vi "Set Modules.vi"(6 "wait for reply (T)":bool=TRUE, 8 "error in (no error)":errorcluster, 10 "Module Paths":path[](array[path])=[path "Modules/Dummie"]) -> (0 "error out":errorcluster, 1 "timed out?":bool)   [LabVIEW 2022 SP3, in "UI Manager.lvlib"]
doc: "Lets UI know which modules are loaded so it can register for broadcast events\n____\nHAMPEL SOFTWARE ENGINEERING v2.6.0 (2023-12-19 10:54)"
uses:
  UI Manager.lvlib
  Set Modules Argument--cluster.ctl
  Set Modules (Reply Payload)--cluster.ctl
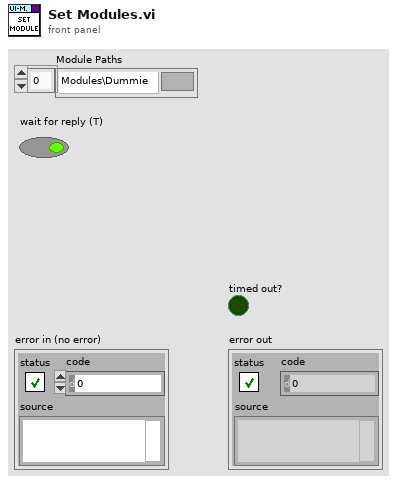
[diagram p1: front panel]
types:
  T1 = typedef "UI Manager.lvlib/Set Modules Argument--cluster.ctl" = cluster{"Module Paths":path[], "Wait Notifier":refnum<notifier>, "wait for reply":bool}
  T2 = typedef "UI Manager.lvlib/Request Events--cluster.ctl" = cluster{"Stop Module":refnum<user-event>, "Show Panel":refnum<user-event>, "Hide Panel":refnum<user-event>, "Get Module Execution Status":refnum<user-event>, "Show Diagram":refnum<user-event>, "Set Run-Time Menu":refnum<user-event>, "Show HSE-ABOUT":refnum<user-event>, "Show PROJECT-ABOUT":refnum<user-event>, "Configure":refnum<user-event>, "Prepare":refnum<user-event>, "Update Status Bar":refnum<user-event>, "Trigger System Message":refnum<user-event>, "Add Module to Run-Time Menu":refnum<user-event>, "Set Modules":refnum<user-event>, "Register for Module Events":refnum<user-event>, "Display another Module UI":refnum<user-event>, "Set Run-Time Menu Visibility":refnum<user-event>, "Set Window Closeable State":refnum<user-event>, "Shutdown Application":refnum<user-event>, "Remove Module from Run-Time Menu":refnum<user-event>, "Set CLI Arguments":refnum<user-event>, "Get CLI Arguments":refnum<user-event>, "External Login":refnum<user-event>, "Get User Level":refnum<user-event>}
  T3 = typedef "UI Manager.lvlib/Set Modules (Reply Payload)--cluster.ctl" = cluster{"error":errorcluster}
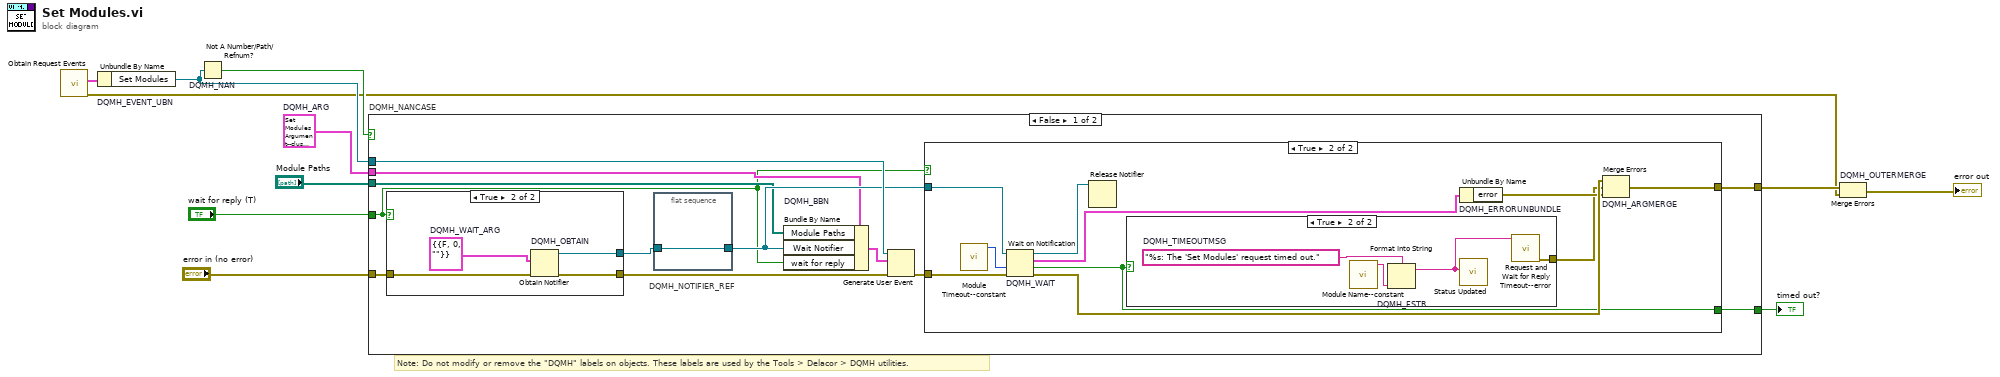
[diagram p0: block diagram]
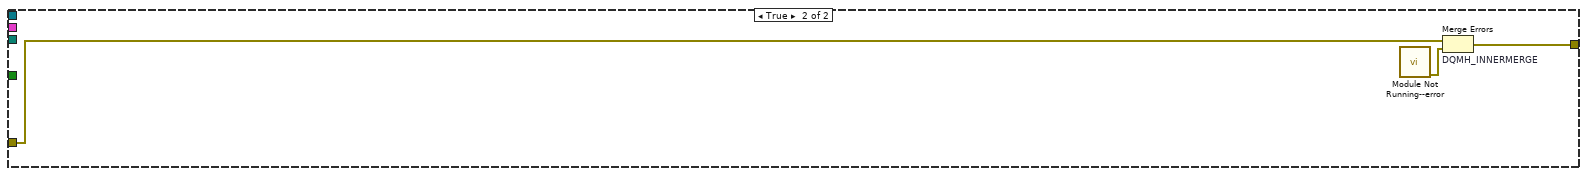
[diagram p5: hidden frame]
diagram:
  w5 = T1 {"Module Paths"=[path "Modules/Dummie"], "Wait Notifier"=refnum, "wait for reply"=FALSE}  # DQMH_ARG
  # "Note: Do not modify or remove the \"DQMH\" labels on objects. These labels are used by the Tools > Delacor > DQMH utilities."
  n1 = call "Obtain Request Events.vi"() -> ("error out"=w2:errorcluster, "UI Manager Request Events"=w1:T2)  [unwired: 10 in]
  n2 = Unbundle By Name "DQMH_EVENT_UBN"(w1) -> ("Set Modules"=w9:refnum<user-event>)
  n3 = Not A Number/Path/Refnum? "DQMH_NAN"(number/path/refnum=w9) -> (NaN/Path/Refnum?=w8:bool)
  n4 = case "DQMH_NANCASE" shown="False" w8 {
    tunnel: "error in (no error)" -> [w23 w47]
    tunnel: w9 -> [w21 _]
    tunnel: [w18 w46] -> w6
    tunnel: [w19 _] -> w7
    tunnel: w5 -> [w14 _]
    tunnel: "Module Paths" -> [w13 _]
    tunnel: "wait for reply (T)" -> [w12 _]
    frame False {
      n5 = case shown="True" w12 {
        tunnel: w23 -> [w40 w44]
        tunnel: [w40 w43] -> w20
        tunnel: [_ w41] -> w16
        frame False {
        }
        frame True {
          w42 = T3 {"error"={"status"=FALSE, "code"=0, "source"=""}}  # DQMH_WAIT_ARG
          n6 = Obtain Notifier "DQMH_OBTAIN"(notification data type=w42, error in (no error)=w44) -> (notifier out=w41:refnum<notifier>, error out=w43:errorcluster)  [unwired: 2 in, 1 out]
        }
      }
      n7 = flat-sequence "DQMH_NOTIFIER_REF" {
        tunnel: w16 -> [w24]
        tunnel: [w24] -> w15
        frame #0 {
        }
      }
      n8 = Bundle By Name "DQMH_BBN"(cluster=w14, "Module Paths"=w13, "Wait Notifier"=w15, "wait for reply"=w12) -> (w17:T1)
      n9 = Generate User Event(user event=w21, event data cluster=w17, error in=w20) -> (error out=w22:errorcluster)  [unwired: 1 in, 1 out]
      n10 = case shown="True" w12 {
        tunnel: w22 -> [w25 w35]
        tunnel: w15 -> [_ w33]
        tunnel: [_ w31] -> w19
        tunnel: [w25 w30] -> w18
        frame False {
        }
        frame True {
          n11 = call "Module Timeout--constant.vi"() -> ("Module Timeout"=w27:i32)  [unwired: 11 in]
          n12 = Wait on Notification "DQMH_WAIT"(notifier=w33, timeout in ms (-1)=w27, error in (no error)=w35) -> (notifier out=w32:refnum<notifier>, notification=w28:T3, timed out?=w31:bool, error out=w34:errorcluster)  [unwired: 1 in]
          n13 = Release Notifier(notifier=w32) -> ()  [unwired: 2 in, 3 out]
          n14 = case shown="True" w31 {
            tunnel: [_ w36] -> w26
            frame False {
            }
            frame True {
              w39 = "%s: The 'Set Modules' request timed out."  # DQMH_TIMEOUTMSG
              n15 = call "Module Name--constant.vi"() -> ("Module Name"=w38:string)  [unwired: 11 in]
              n16 = Format Into String "DQMH_FSTR"(format string=w39, w38) -> (resulting string=w37:string)  [unwired: 2 in, 1 out]
              n17 = call "Status Updated.vi"("Status"=w37) -> ()  [unwired: 10 in, 1 out]
              n18 = call "Request and Wait for Reply Timeout--error.vi"("Error Message"=w37) -> ("error out"=w36:errorcluster)  [unwired: 10 in]
            }
          }
          n19 = Unbundle By Name "DQMH_ERRORUNBUNDLE"(w28) -> ("error"=w29:errorcluster)
          n20 = Merge Errors "DQMH_ARGMERGE"(w34, w26, w29) -> (w30:errorcluster)
        }
      }
    }
    frame True {
      n21 = call "Module Not Running--error.vi"() -> ("error out"=w45:errorcluster)  [unwired: 11 in]
      n22 = Merge Errors "DQMH_INNERMERGE"(w47, w45) -> (w46:errorcluster)
    }
  }
  "timed out?" <- w7
  n23 = Merge Errors "DQMH_OUTERMERGE"(w6, w2) -> (→"error out":errorcluster)
